vi "Digital Integrator Reset.vi"(8 "error in (no error)":errorcluster, 10 "Gain":i16(slide)=1 min=0 max=9 step=1 scale=0.0..9.0, 11 "VISA resource name":refnum<visa-resource-name>) -> (3 "VISA resource name":refnum<visa-resource-name>)   [LabVIEW 2025]
doc: "Author: Scott Hannahs <sth@magnet.fsu.edu>\n\nThis software is licensed for use under the “MIT License\"\nCopyright (c) 2025 Scott Hannahs, sth@sth@magnet.sthnet.net\n\nPermission is hereby granted, free of charge, to any person obtaining a copy of this software and associated documentation files (the \"Software\"), to deal in the Software without restriction, including without limitation the rights to use, copy, modify, merge, publish, distribute, sublicense, and/or sell copies of the Software, and to permit persons to whom the Software is furnished to do so, subject to the following conditions: The above copyright notice and this permission notice shall be included in all copies or substantial portions of the Software.\n\nTHE SOFTWARE IS PROVIDED \"AS IS\", WITHOUT WARRANTY OF ANY KIND, EXPRESS OR IMPLIED, INCLUDING BUT NOT LIMITED TO THE WARRANTIES OF MERCHANTABILITY, FITNESS FOR A PARTICULAR PURPOSE AND NONINFRINGEMENT. IN NO EVENT SHALL THE AUTHORS OR COPYRIGHT HOLDERS BE LIABLE FOR ANY CLAIM, DAMAGES OR OTHER LIABILITY, WHETHER IN AN ACTION OF CONTRACT, TORT OR OTHERWISE, ARISING FROM, OUT OF OR IN CONNECTION WITH THE SOFTWARE OR THE USE OR OTHER DEALINGS IN THE SOFTWARE."
panel:
  out "error out":errorcluster
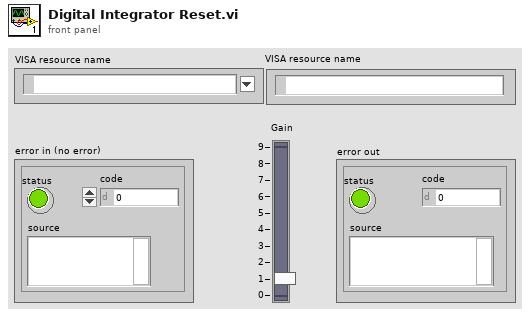
[diagram p1: front panel]
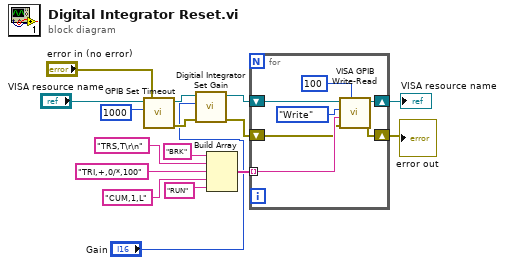
[diagram p0: block diagram]
diagram:
  n1 = call "GPIB Set Timeout.vi"("Error In"="error in (no error)", "Timeout"=u32 1000, "VISA resource name"="VISA resource name") -> ("Error Out"=w3:errorcluster, "dup VISA resource name"=w5:refnum<visa-resource-name>)  [unwired: 2 in, 1 out]
  n2 = call "Digitial Integrator Set Gain.vi"("error in (no error)"=w3, "Gain"="Gain", "VISA resource name"=w5) -> ("error out"=w2:errorcluster, "VISA resource name dup"=w4:refnum<visa-resource-name>)  [unwired: 7 in]
  n3 = Build Array("BRK", "TRS,T\r\n", "TRI,+,0/*,100", "CUM,1,L", "RUN") -> (w8:string[])
  n4 = for {
    tunnel: w8 -> [w21] mode=indexing
    shift-right: [w20] -> w14
    shift-left: w4 -> [w23]
    shift-right: [w17] -> w6
    shift-left: w2 -> [w18]
    n5 = call "VISA GPIB Write-Read.vi"("Wait (ms)"=u32 100 ("wait (mS)"), "error in (no error)"=w18, "Command"=w21, "Action"=enum16{"Write", "Read", "Write & Read"}."Write", "VISA resource name"=w23) -> ("error out"=w17:errorcluster, "dup VISA Session"=w20:refnum<visa-resource-name>)  [unwired: 3 in, 2 out]
  }
  "VISA resource name" <- w14
  "error out" <- w6
